vi "Initialize.vi"(7 "Serial Configuration":T1={"Baud Rate"=9600, "Parity"=0, "Data Bits"=8, "Stop Bits"=10, "Flow Control"=0} {"Flow Control" items=["None", "XON/XOFF", "RTS/CTS", "XON/XOFF & RTS/CTS", "DTR/DSR", "XON/XOFF & DTR/DSR"]; "Stop Bits" items=["1.0"=10, "1.5"=15, "2.0"=20]; "Data Bits" items=["8"=8]; "Parity" items=["None", "Odd", "Even", "Mark", "Space"]; "Baud Rate" items=["300"=300, "600"=600, "1200"=1200, "2400"=2400, "4800"=4800, "9600"=9600, "19200"=19200]}, 8 "error in (no error)":errorcluster, 9 "Reset (True)":bool=TRUE, 10 "ID Query (True)":bool=TRUE, 11 "VISA resource name":refnum<visa-resource-name>) -> (0 "error out":errorcluster, 3 "VISA resource name out":refnum<visa-resource-name>)   [LabVIEW 2021, in "BK Precision 5491B.lvlib"]
doc: "Establishes communication with the instrument and optionally performs an instrument identification query and/or an instrument reset. It also places the instrument in a default state needed for other instrument driver operations. Therefore, call this VI before calling other instrument driver VIs for this instrument. Generally, you need to call the <b>Initialize</b> VI only once at the beginning of an application."
uses:
  <instrlib>/BK Precision 5491B/BK Precision 5491B.lvlib
panel:
  # "(c) 2016 B&K Precision Corporation.  ALL RIGHTS RESERVED."
  # "NOTE: Before initializing connection to the instrument, go into the instrument system menu and set TX TERM to LF and RETURN to OFF."
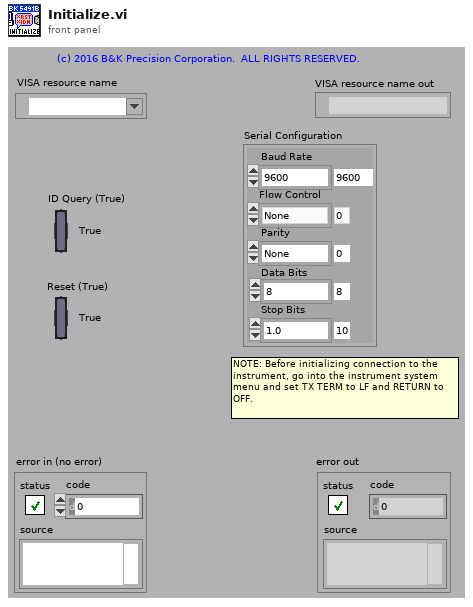
[diagram p1: front panel]
types:
  T1 = cluster{"Baud Rate":u32, "Parity":u16, "Data Bits":u16, "Stop Bits":u16, "Flow Control":u16}
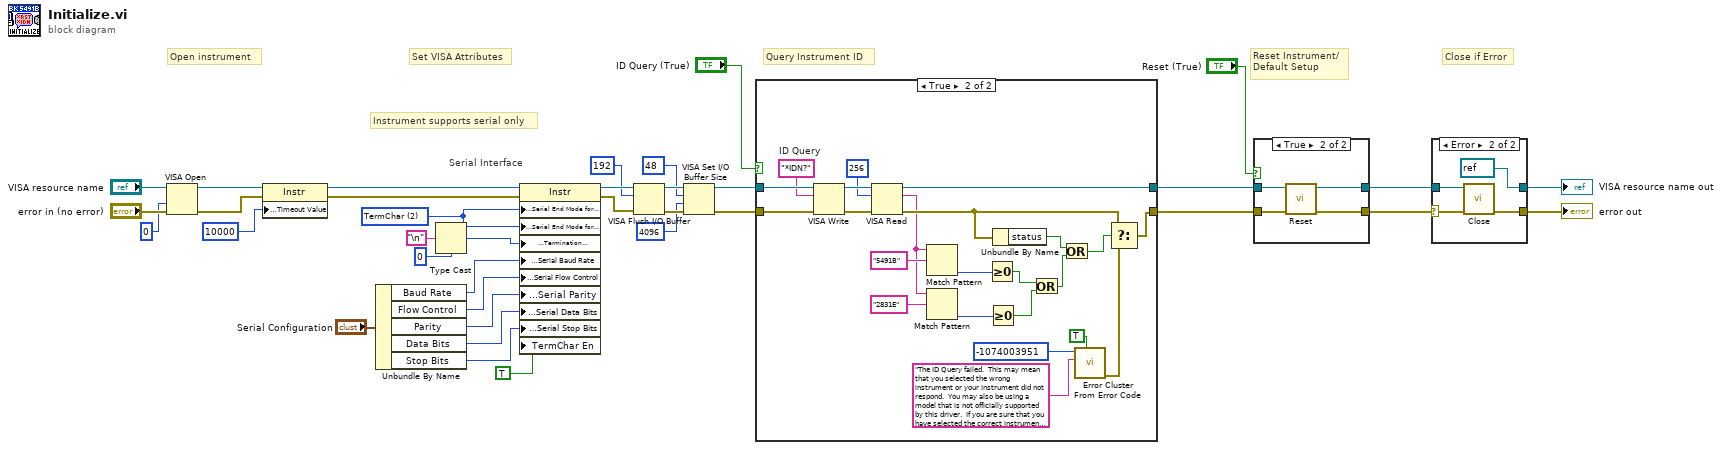
[diagram p0: block diagram]
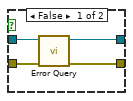
[diagram p3: hidden frame]
diagram:
  w11 = u16 2 items=["None", "LastBit", "TermChar"] ("Serial Settings:Serial End Mode for Reads")
  # "Instrument supports serial only"
  # "Serial Interface"
  # "Set VISA Attributes"
  # "Close if Error"
  # "Query Instrument ID"
  # "Reset Instrument/\nDefault Setup"
  # "Open instrument"
  n1 = VISA Open(access mode=u32 0, error in (no error)="error in (no error)", VISA resource name="VISA resource name") -> (VISA resource name=w21:refnum<visa-resource-name>, error out=w22:errorcluster)  [unwired: 2 in]
  n2 = property class="Instr"(reference=w21, error in=w22, "General Settings:Timeout Value"=u32 10000) -> (reference out=w29:refnum<visa-resource-name>, error out=w28:errorcluster)
  n3 = Unbundle By Name("Serial Configuration") -> ("Baud Rate"=w9:u32, "Flow Control"=w5:u16, "Parity"=w7:u16, "Data Bits"=w8:u16, "Stop Bits"=w4:u16)
  n4 = Type Cast(type=u8 0, x="\n" ("Line Feed Constant")) -> (*(type *) &x=w10:u8)
  n5 = property class="Instr"(reference=w29, error in=w28, "Serial Settings:Serial End Mode for Reads"=w11, "Serial Settings:Serial End Mode for Writes"=w11, "Message Based Settings:Termination Character"=w10, "Serial Settings:Serial Baud Rate"=w9, "Serial Settings:Serial Flow Control"=w5, "Serial Settings:Serial Parity"=w7, "Serial Settings:Serial Data Bits"=w8, "Serial Settings:Serial Stop Bits"=w4, "TermChar En"=TRUE ("Message Based Settings:Termination Character Enable")) -> (reference out=w17:refnum<visa-resource-name>, error out=w19:errorcluster)
  n6 = VISA Flush I/O Buffer(VISA resource name=w17, mask (16)=u16 192, error in (no error)=w19) -> (VISA resource name out=w20:refnum<visa-resource-name>, error out=w18:errorcluster)
  n7 = VISA Set I/O Buffer Size(VISA resource name=w20, mask (16)=u16 48, size (4096)=u32 4096 ("size (0)"), error in (no error)=w18) -> (VISA resource name out=w31:refnum<visa-resource-name>, error out=w30:errorcluster)
  n8 = case shown="True" "ID Query (True)" {
    tunnel: [w37 w61] -> w1
    tunnel: [w38 w58] -> w2
    tunnel: w31 -> [w38 w59]
    tunnel: w30 -> [w37 w60]
    frame False {
    }
    frame True {
      w53 = "*IDN?"  # ID Query
      n9 = VISA Write(VISA resource name=w59, write buffer=w53, error in (no error)=w60) -> (VISA resource name out=w57:refnum<visa-resource-name>, error out=w56:errorcluster)  [unwired: 1 out]
      n10 = VISA Read(VISA resource name=w57, byte count=u32 256, error in (no error)=w56) -> (VISA resource name out=w58:refnum<visa-resource-name>, read buffer=w43:string, error out=w47:errorcluster)  [unwired: 1 out]
      n11 = Match Pattern(string=w43, regular expression="5491B") -> (offset past match=w48:i32)  [unwired: 1 in, 3 out]
      n12 = Match Pattern(string=w43, regular expression="2831E") -> (offset past match=w42:i32)  [unwired: 1 in, 3 out]
      n13 = Greater Or Equal To 0?(x=w48) -> (x >= 0?=w41:bool)
      n14 = Greater Or Equal To 0?(x=w42) -> (x >= 0?=w40:bool)
      n15 = Unbundle By Name(w47) -> ("status"=w46:bool)
      n16 = Or(x=w41, y=w40) -> (x .or. y?=w39:bool)
      n17 = Or(x=w46, y=w39) -> (x .or. y?=w45:bool)
      n18 = call <vilib>:"Error Cluster From Error Code.vi"("show call chain? (False)"=TRUE, "error message (\"\")"="The ID Query failed.  This may mean that you selected the wrong instrument or your instrument did not respond.  You may also be using a model that is not officially supported by this driver.  If you are sure that you have selected the correct instrument and it is responding, try disabling the ID Query." ("Source (VI Name)"), "error code (0)"=-1074003951 ("Code")) -> ("error out"=w52:errorcluster)  [unwired: 6 in]
      n19 = Select(t=w47, s=w45, f=w52) -> (s? t:f=w61:errorcluster)
    }
  }
  n20 = case shown="True" "Reset (True)" {
    tunnel: w1 -> [w62 w66]
    tunnel: [w64 w69] -> w23
    tunnel: w2 -> [w63 w67]
    tunnel: [w65 w68] -> w24
    frame False {
      n21 = call <instrlib>:"Error Query.vi"("error in (no error)"=w62, "VISA resource name"=w63) -> ("error out"=w64:errorcluster, "VISA resource name out"=w65:refnum<visa-resource-name>)  [unwired: 7 in, 1 out]
    }
    frame True {
      n22 = call <instrlib>:"Reset.vi"("error in (no error)"=w66, "VISA resource name"=w67) -> ("error out"=w69:errorcluster, "VISA resource name out"=w68:refnum<visa-resource-name>)  [unwired: 8 in]
    }
  }
  n23 = case shown="Error" w23 {
    selector: w23 -> [w70 w73]
    tunnel: w24 -> [w71 w74]
    tunnel: [w71 refnum<visa-resource-name> refnum ("VISA resource name out")] -> w26
    tunnel: [w70 w75] -> w25
    frame No Error {
    }
    frame Error {
      n24 = call <instrlib>:"Close.vi"("error in (no error)"=w73, "VISA resource name"=w74) -> ("error out"=w75:errorcluster)  [unwired: 9 in]
    }
  }
  "VISA resource name out" <- w26
  "error out" <- w25
